vi "BRig_RT__Case_Exp__UploadClosedLoop_getFirstCmd.vi"(11 "input_str":string) -> (0 "output_cmd":string, 1 "output_cmd":bool, 3 "output_str":string, 5 "output_abort":bool)   [LabVIEW 2014]
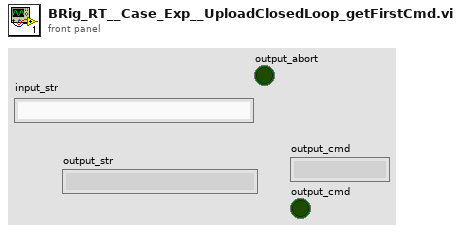
[diagram p1: front panel]
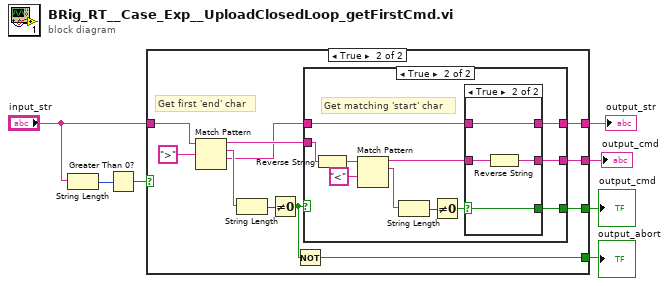
[diagram p0: block diagram]
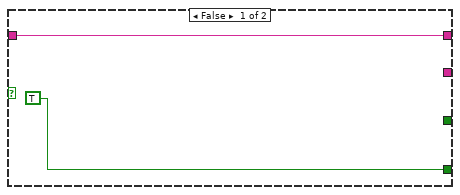
[diagram p2: hidden frame]
diagram:
  n1 = String Length(string="input_str") -> (length=w7:i32)
  n2 = Greater Than 0?(x=w7) -> (x > 0?=w6:bool)
  n3 = case shown="True" w6 {
    tunnel: "input_str" -> [w9 w19]
    tunnel: [w9 w17] -> w4
    tunnel: [_ w13] -> w3
    tunnel: [_ w12] -> w2
    tunnel: [TRUE w10] -> w1
    frame False {
    }
    frame True {
      # "Get first 'end' char"
      n4 = Match Pattern(string=w19, regular expression=">" ("search string/char (-)")) -> (before substring=w15:string, match substring=w16:string, after substring=w14:string)  [unwired: 1 in, 1 out]
      n5 = String Length(string=w16) -> (length=w18:i32)
      n6 = Not Equal To 0?(x=w18) -> (x != 0?=w11:bool)
      n7 = Not(x=w11) -> (.not. x?=w10:bool)
      n8 = case shown="True" w11 {
        tunnel: w15 -> [w21 w30]
        tunnel: [w21 w26] -> w17
        tunnel: w14 -> [_ w24]
        tunnel: [_ w23] -> w13
        tunnel: [_ w22] -> w12
        frame False {
        }
        frame True {
          # "Get matching 'start' char"
          n9 = Reverse String(1:w30) -> (0:w31:string)
          n10 = Match Pattern(string=w31, regular expression="<") -> (before substring=w25:string, match substring=w28:string)  [unwired: 1 in, 2 out]
          n11 = String Length(string=w28) -> (length=w29:i32)
          n12 = Not Equal To 0?(x=w29) -> (x != 0?=w27:bool)
          n13 = case shown="True" w27 {
            selector: w27 -> [_ w34]
            tunnel: w25 -> [_ w36]
            tunnel: [w33 w37] -> w26
            tunnel: w24 -> [w33 w37]
            tunnel: [_ w35] -> w23
            tunnel: [_ w34] -> w22
            frame False {
            }
            frame True {
              n14 = Reverse String(1:w36) -> (0:w35:string)
            }
          }
        }
      }
    }
  }
  "output_str" <- w4
  "output_cmd" <- w3
  "output_cmd" <- w2
  "output_abort" <- w1
